vi "Number of Clusters With Silhouette Analysis.vi"() -> ()   [LabVIEW 2020]
doc: "Silhouette analysis can be used to study the separation distance between the resulting clusters. The silhouette plot displays a measure of how close each point in one cluster is to points in the neighboring clusters and thus provides a way to assess parameters like number of clusters visually. This measure has a range of [-1, 1].\n\nSilhouette coefficients (as these values are referred to as) near +1 indicate that the sample is far away from the neighboring clusters. A value of 0 indicates that the sample is on or very close to the decision boundary between two neighboring clusters and negative values indicate that those samples might have been assigned to the wrong cluster.\n\nIn this example the silhouette analysis is used to choose an optimal value for n_clusters. The silhouette plot shows that the n_clusters value of 3, 5 and 6 are a bad pick for the given data due to the presence of clusters with below average silhouette scores and also due to wide fluctuations in the size of the silhouette plots. Silhouette analysis is more ambivalent in deciding between 2 and 4.\n\nAlso from the thickness of the silhouette plot the cluster size can be visualized. The silhouette plot for cluster 0 when n_clusters is equal to 2, is bigger in size owing to the grouping of the 3 sub clusters into one big cluster. However when the n_clusters is equal to 4, all the plots are more or less of similar thickness and hence are of similar sizes as can be also verified from the labelled scatter plot on the right."
uses:
  Model/Unsupervised/Cluster/KMeans/Controls/kmeans_params.ctl
  Display/_Controls/Style.ctl
  Display/Classification/2D/Predicted/Controls/PredictedParameter.ctl
  Model/Unsupervised/Cluster/KMeans/KMeans.lvclass
  C:/Users/cipop/TDF Dropbox/2_Technologies de France/1 - Services et Etudes/PLAIY/2 - DEV/PLAIYLAB/code/Model/Model.lvclass
  Model/Unsupervised/Cluster/KMeans/KMeans.vi
  Preproc/Objet/3 - Model selection and evaluation/3.3 - Metrics and scoring/silhouette_score/Silhouette_Score.vi
  Preproc/Objet/3 - Model selection and evaluation/3.3 - Metrics and scoring/silhouette_samples/Silhouette_Samples.vi
panel:
  out "XY Graph 10":cluster{"X":dbl[], "Y":dbl[]}[](graph)
  out "XY Graph 9":cluster{"X":dbl[], "Y":dbl[]}[](graph)
  out "XY Graph 8":cluster{"X":dbl[], "Y":dbl[]}[](graph)
  out "XY Graph 7":cluster{"X":dbl[], "Y":dbl[]}[](graph)
  out "XY Graph 6":cluster{"X":dbl[], "Y":dbl[]}[](graph) caption="The visualization of the clustered data"
  out "XY Graph 5":cluster{"X":dbl[], "Y":dbl[]}[](graph)
  out "XY Graph 4":cluster{"X":dbl[], "Y":dbl[]}[](graph)
  out "XY Graph 3":cluster{"X":dbl[], "Y":dbl[]}[](graph)
  out "XY Graph 2":cluster{"X":dbl[], "Y":dbl[]}[](graph)
  out "XY Graph":cluster{"X":dbl[], "Y":dbl[]}[](graph) caption="The silhouette plot for the various clusters"
  out "silhouette_avg":string[](array[string])
  in  "Local":T1
  out "error out":errorcluster
  in  "error in":errorcluster
  # "Silhouette analysis for KMeans clustering on sample data with n_cluster = 2"
  # "Silhouette analysis for KMeans clustering on sample data with n_cluster = 3"
  # "Silhouette analysis for KMeans clustering on sample data with n_cluster = 4"
  # "Silhouette analysis for KMeans clustering on sample data with n_cluster = 5"
  # "Silhouette analysis for KMeans clustering on sample data with n_cluster = 6"
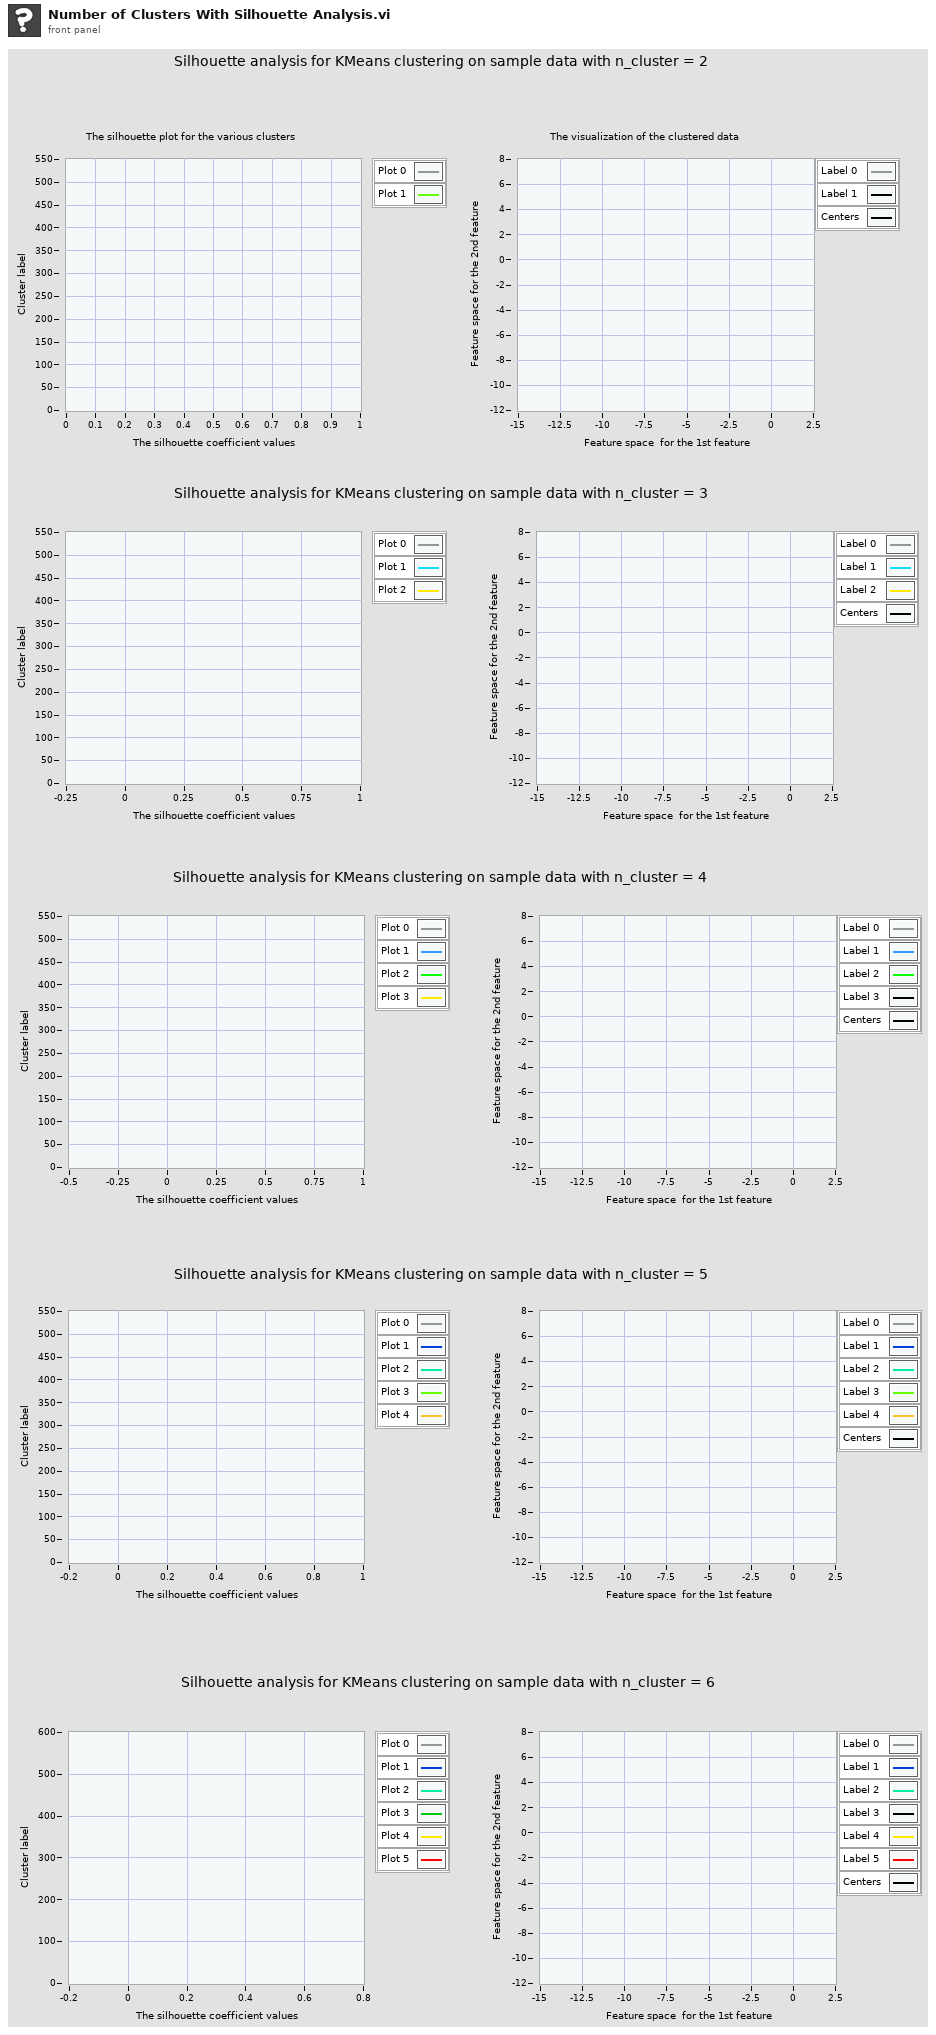
[diagram p1: front panel]
types:
  T1 = cluster{"X":dbl[][], "cluster_labels":dbl[][][], "cluster_centers_":dbl[][][], "sample_silhouette_values":dbl[][], "range_n_clusters":i32[], "ith_cluster_silhouette_values":cluster{"X":dbl[]}[], "y":cluster{"y":dbl[]}[], "i":i32[][][], "Silhouette Plot":refnum<vi>[], "Clustered Plot":refnum<vi>[]}
  T2 = cluster{"n_samples":i32[], "n_features":u32, "centers":i32[][], "cluster_std":dbl[], "centermin":dbl, "centermax":dbl, "shuffle":bool, "random_state":i32, "Returns":string}
  T3 = typedef "kmeans_params.ctl" = cluster{"n_clusters":dbl, "init":cluster{"init_type":string, "init_list":dbl[][]}, "n_init":dbl, "max_iter":dbl, "tol":dbl, "verbose":dbl, "random_state":dbl, "copy_x":bool, "algorithm":string}
  T4 = typedef "Style.ctl" = enum16{"Empty circle", "Full circle", "Empty square", "Full square", "Cross"}
  T5 = typedef "PredictedParameter.ctl" = cluster{"Plot":refnum<vi>, "Data":cluster{"X":dbl[][], "Predict":dbl[][]}, "Indexe":cluster{"X":i32, "Y":i32}, "Point Property":cluster{"Style":T4, "Label Color":u32[]}}
  T6 = cluster{" 4DArray":cluster{"1":string[][], "2":string[][]}[], " 3DArray":cluster{"Tableau":string[][]}[], "Sparse Matrix 2DArray":string[][], " 2DArray":string[][], " 1DArray":string[]}
  T7 = typedef "kmeans_attributes.ctl" = cluster{"cluster_centers_":dbl[][], "labels_":dbl[], "inertia_":dbl, "n_iter_":dbl}
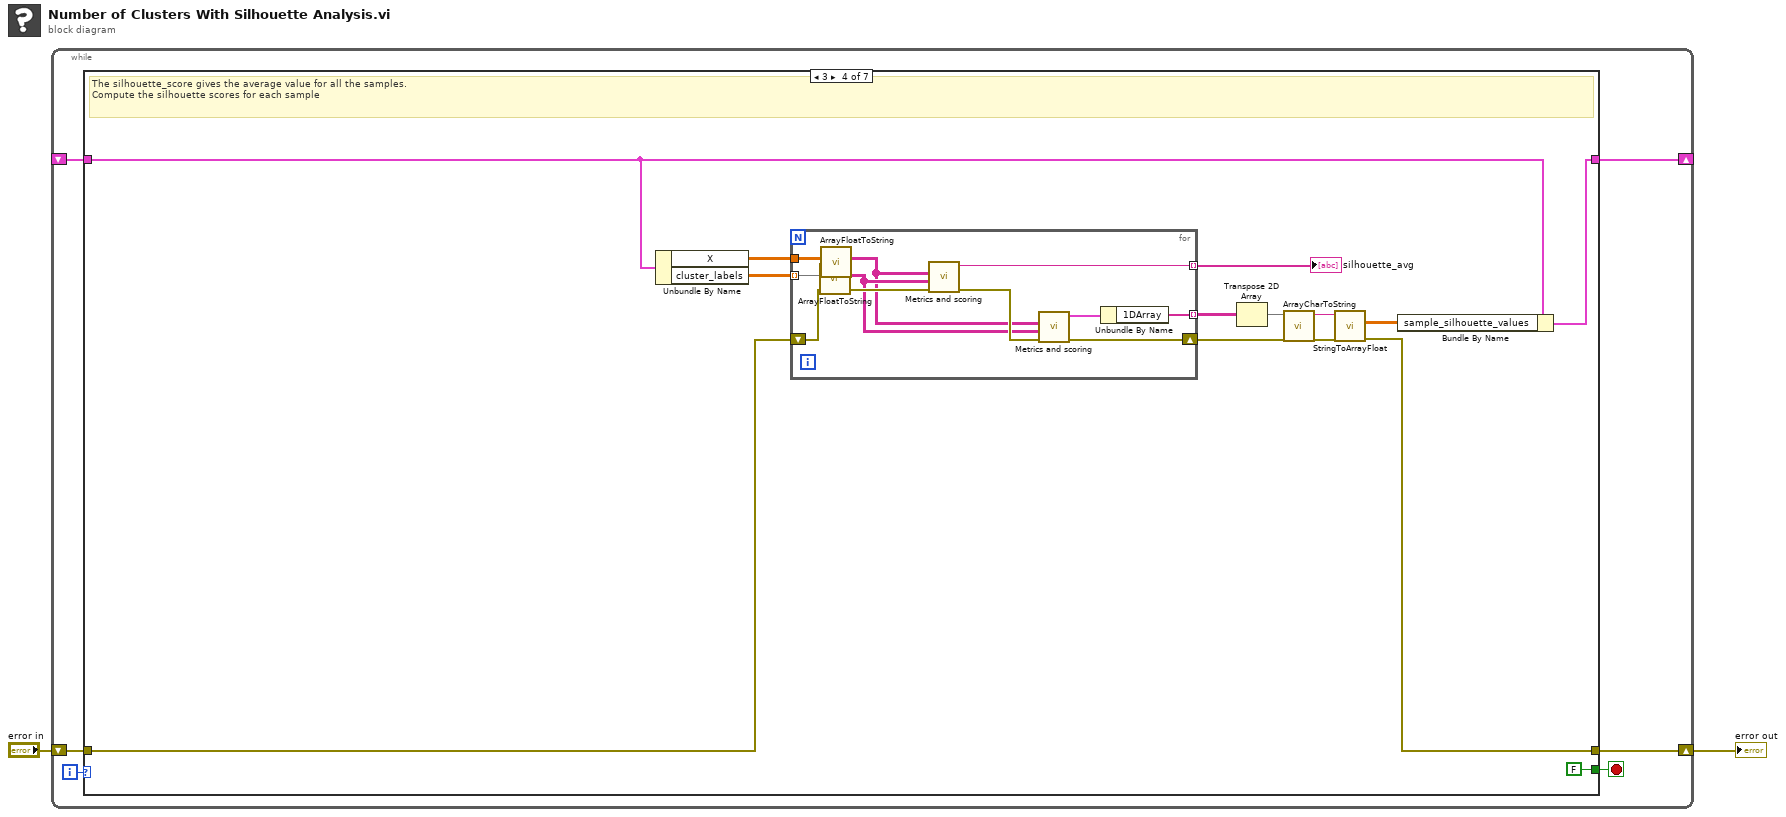
[diagram p0: block diagram]
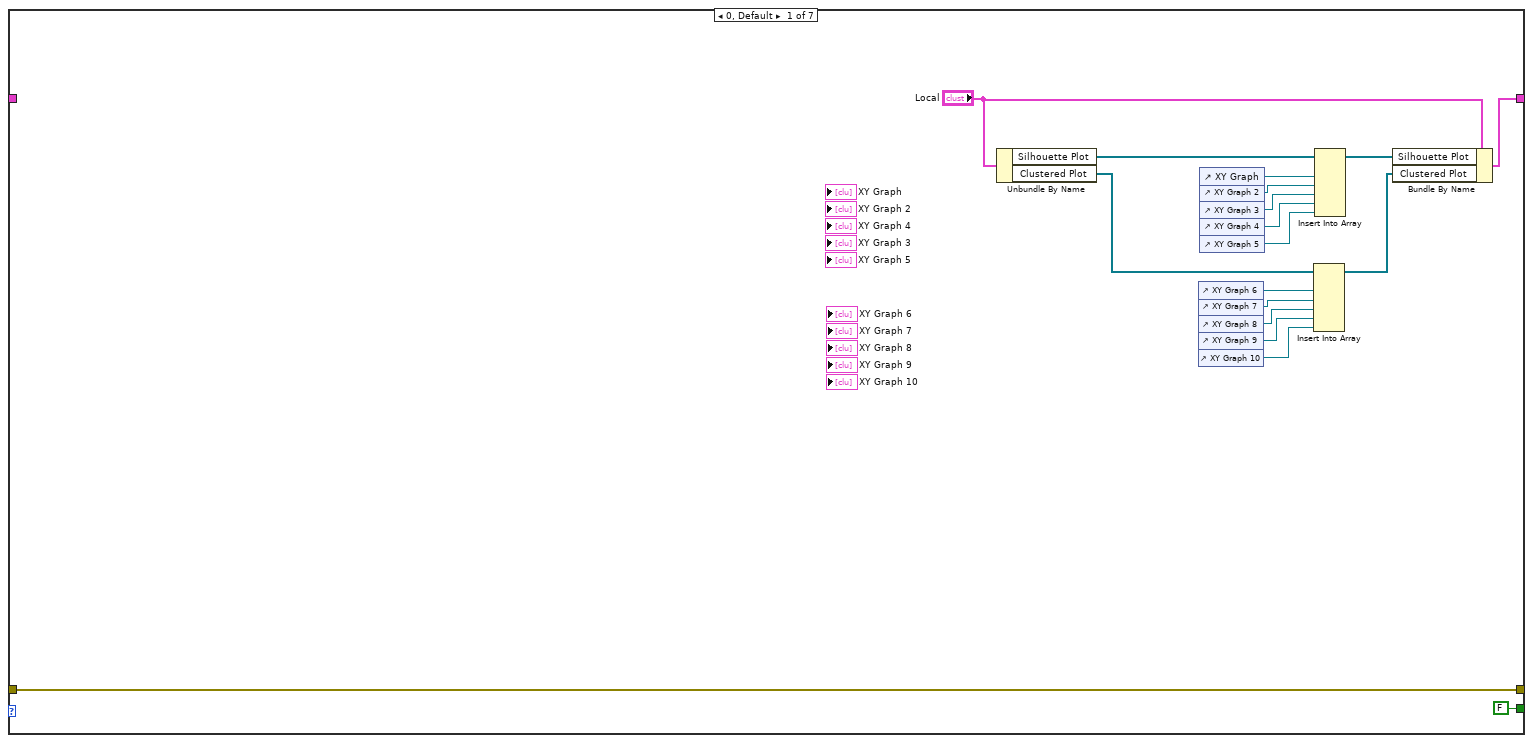
[diagram p2: hidden frame]
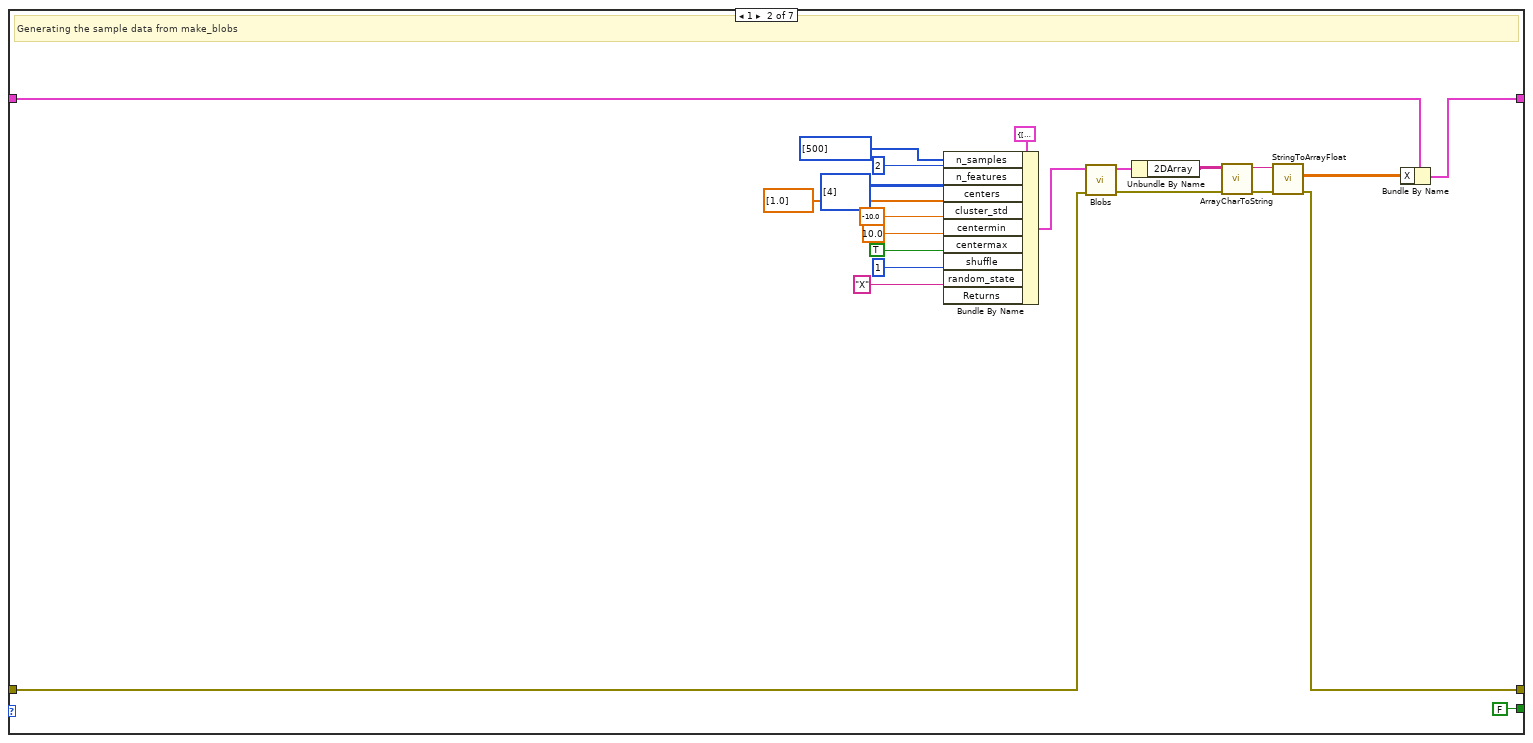
[diagram p3: hidden frame]
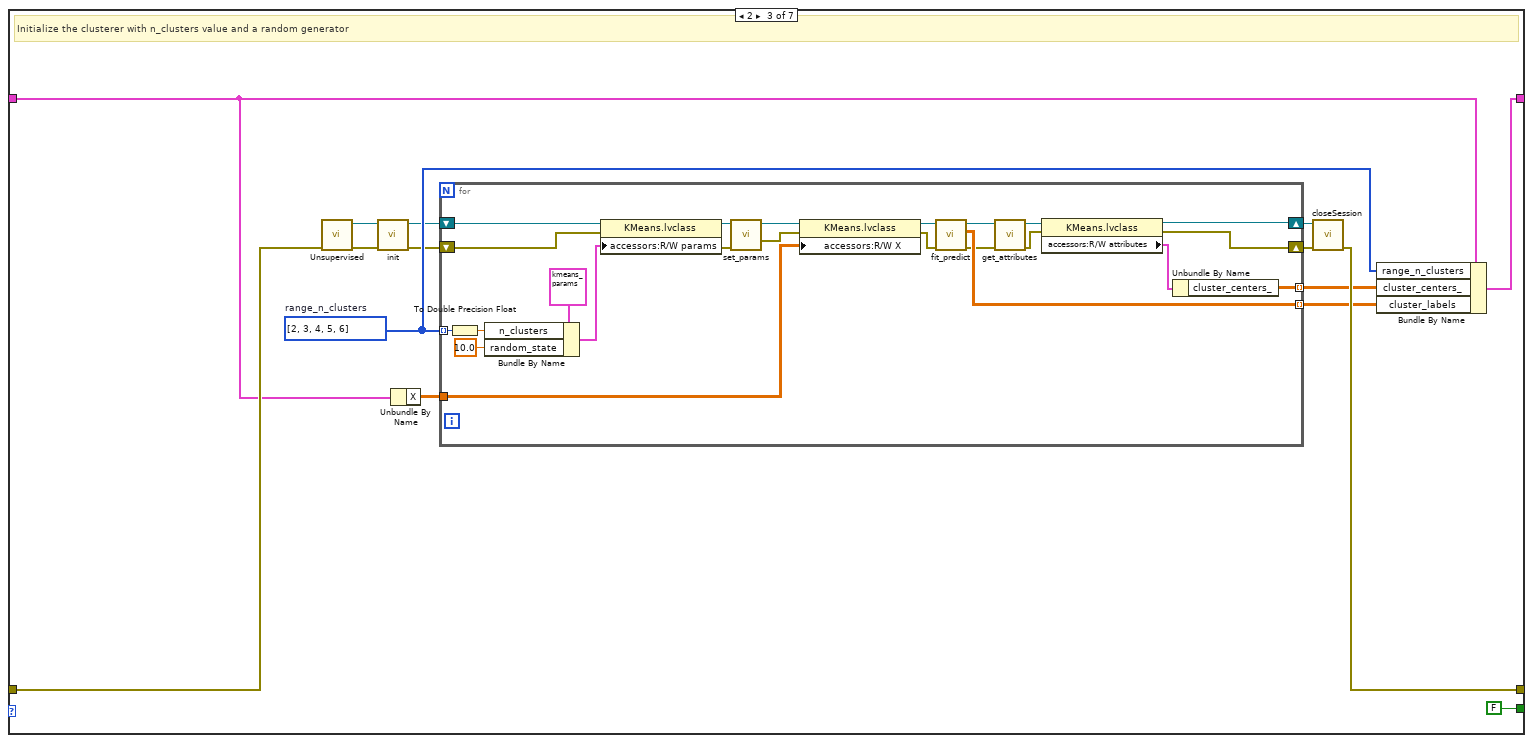
[diagram p4: hidden frame]
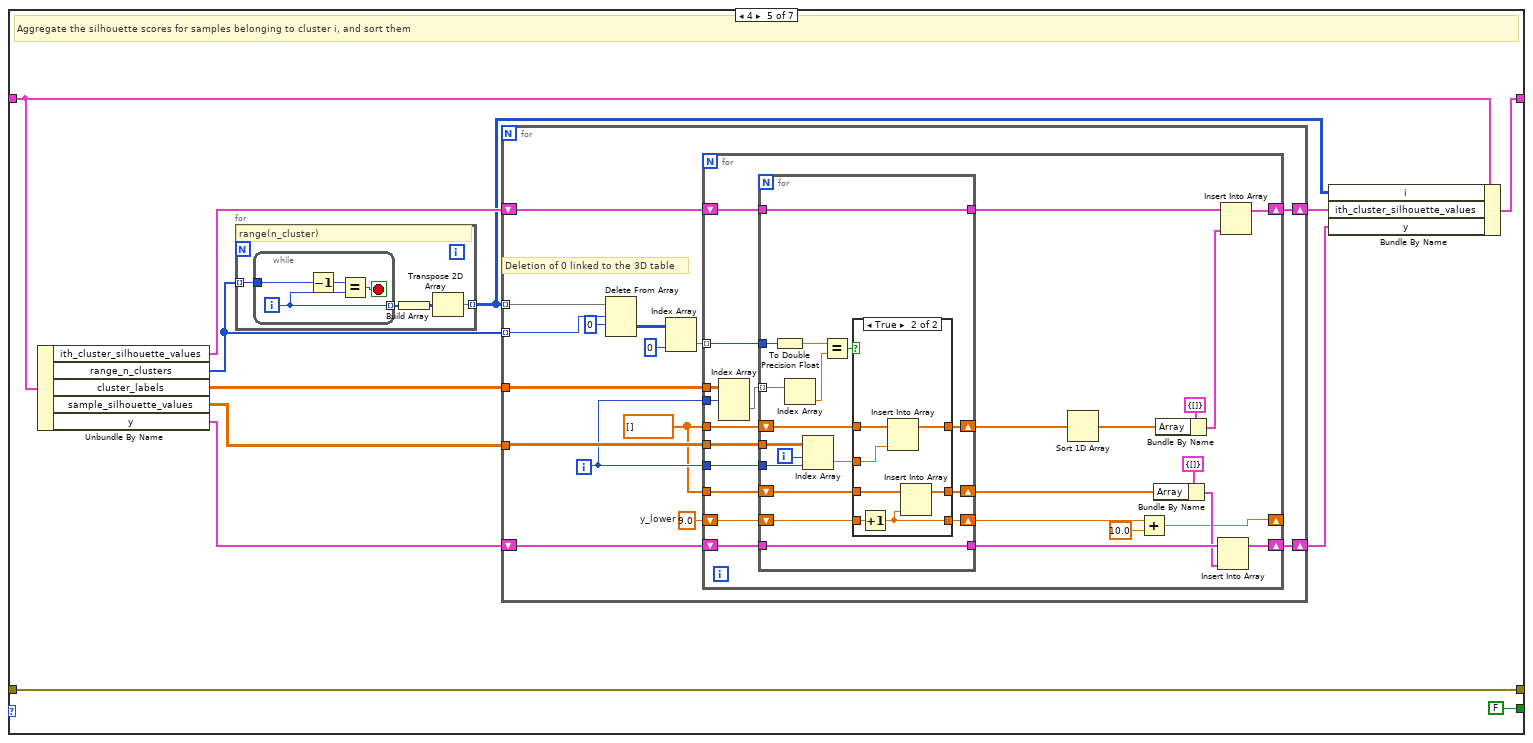
[diagram p5: hidden frame]
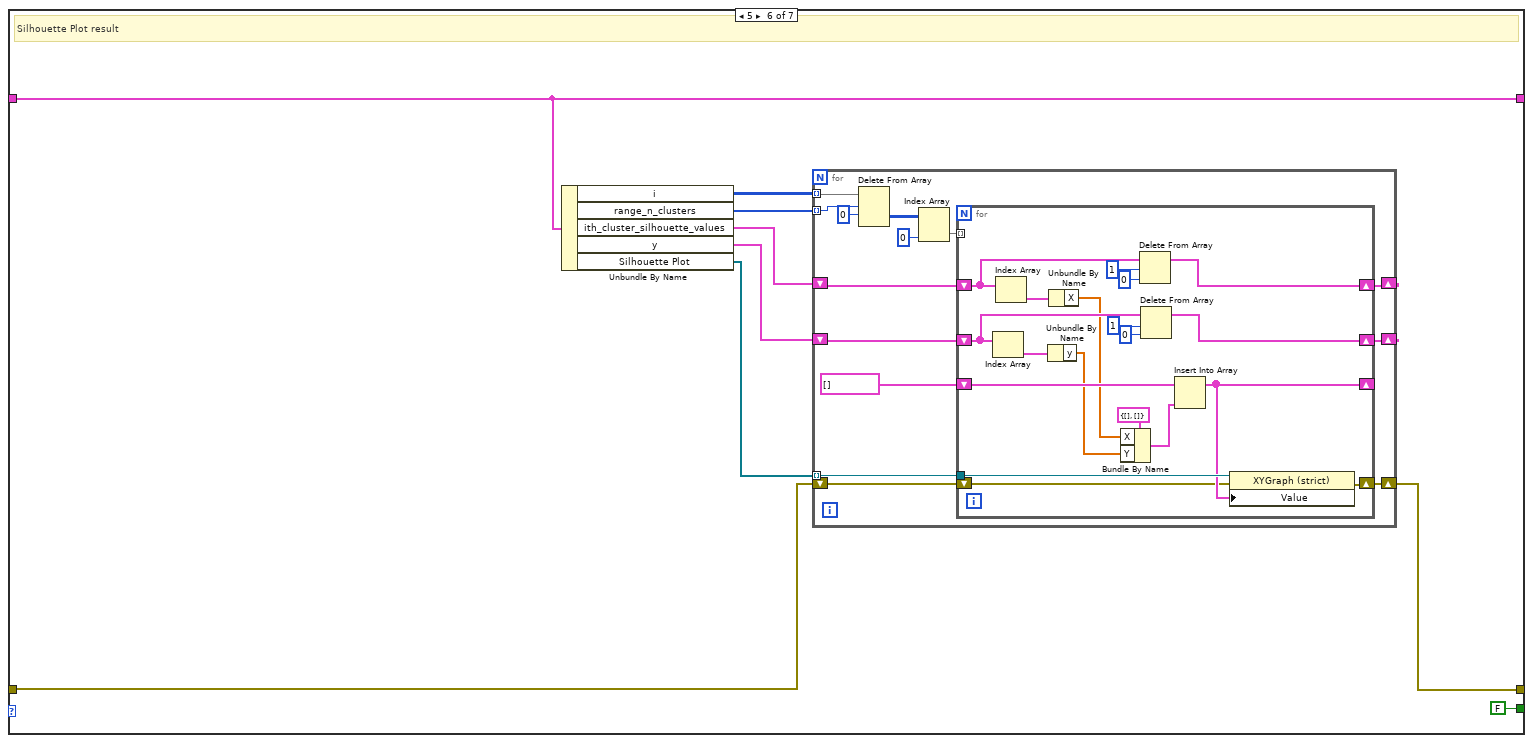
[diagram p7: hidden frame]
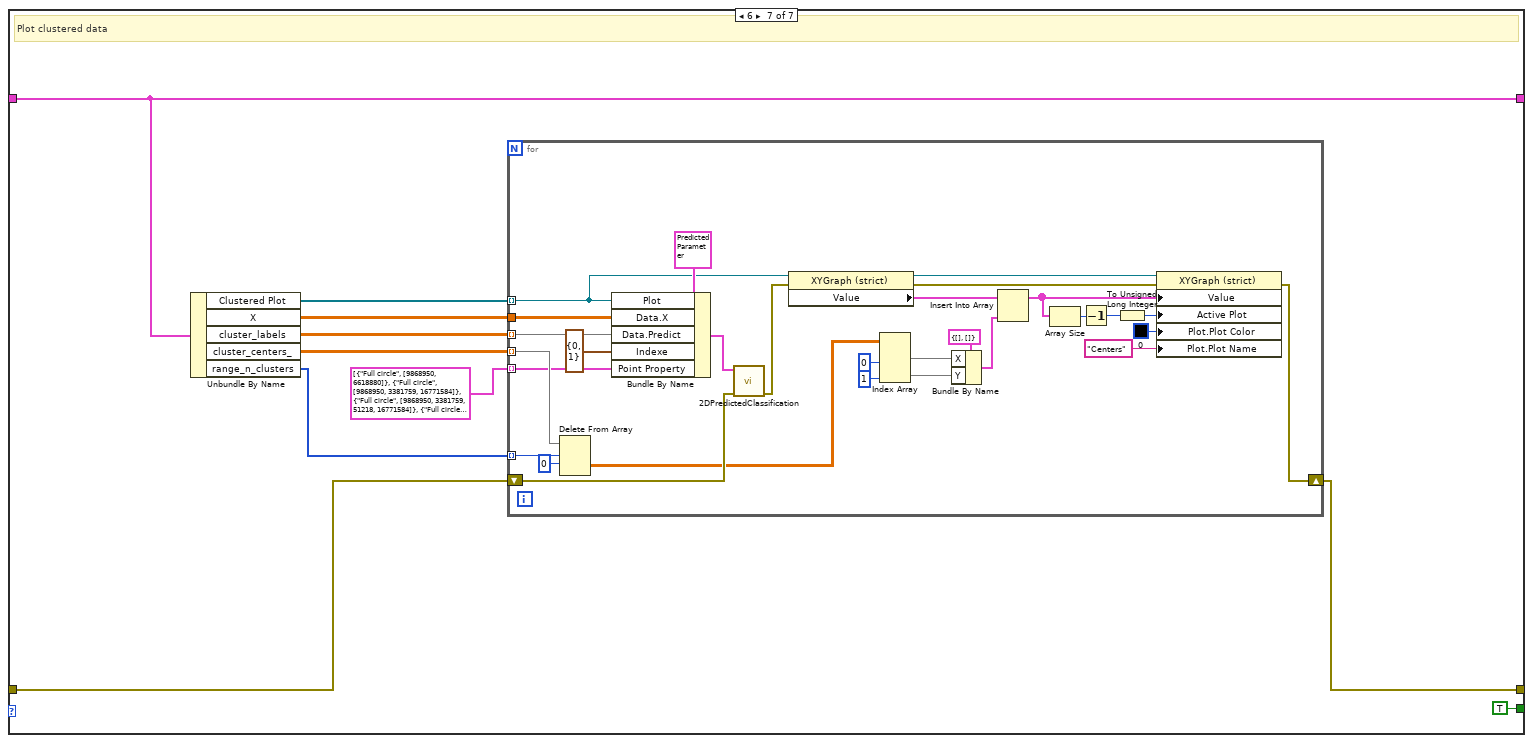
[diagram p8: hidden frame]
diagram:
  n1 = while {
    shift-right: [w6] -> w1
    shift-left: "error in" -> [w7]
    shift-right: [w5] -> _
    shift-left: _ -> [w4]
    i -> [w8]
    stop <- w3 stop-if-true
    n2 = case shown="3" w8 {
      tunnel: w7 -> [w26 w34 w62 w98 w119 w198 w241]
      tunnel: [w26 w33 w61 w94 w119 w197 w240] -> w6
      tunnel: [w21 w31 w59 w95 w113 w203 w246] -> w5
      tunnel: w4 -> [_ w32 w49 w96 w112 w203 w246]
      tunnel: [FALSE FALSE FALSE FALSE FALSE FALSE TRUE] -> w3
      frame 0, Default {
        n3 = Unbundle By Name("Local") -> ("Silhouette Plot"=w23:refnum<vi>[], "Clustered Plot"=w15:refnum<vi>[])
        n4 = control-ref of="XY Graph 6"() -> (w13:refnum<vi>)
        n5 = control-ref of="XY Graph 7"() -> (w12:refnum<vi>)
        n6 = control-ref of="XY Graph 8"() -> (w11:refnum<vi>)
        n7 = control-ref of="XY Graph 9"() -> (w10:refnum<vi>)
        n8 = control-ref of="XY Graph 10"() -> (w9:refnum<vi>)
        n9 = control-ref of="XY Graph"() -> (w20:refnum<vi>)
        n10 = control-ref of="XY Graph 2"() -> (w19:refnum<vi>)
        n11 = control-ref of="XY Graph 3"() -> (w18:refnum<vi>)
        n12 = control-ref of="XY Graph 4"() -> (w17:refnum<vi>)
        n13 = control-ref of="XY Graph 5"() -> (w16:refnum<vi>)
        n14 = Insert Into Array(array=w15, new element #1=w13, new element #2=w12, new element #3=w11, new element #4=w10, new element #5=w9) -> (w14:refnum<vi>[])  [unwired: 1 in]
        n15 = Insert Into Array(array=w23, new element #1=w20, new element #2=w19, new element #3=w18, new element #4=w17, new element #5=w16) -> (w22:refnum<vi>[])  [unwired: 1 in]
        n16 = Bundle By Name(cluster="Local", "Silhouette Plot"=w22, "Clustered Plot"=w14) -> (w21:T1)
      }
      frame 1 {
        # "Generating the sample data from make_blobs"
        n17 = Bundle By Name(cluster=T2 {"n_samples"=[100], "n_features"=2, "centers"=[], "cluster_std"=[1.0], "centermin"=-10.0, "centermax"=10.0, "shuffle"=TRUE, "random_state"=-1, "Returns"="X"} ("make_blobs"), "n_samples"=i32[] [500], "n_features"=u32 2, "centers"=i32[][] [[4]], "cluster_std"=dbl[] [1.0], "centermin"=-10.0, "centermax"=10.0, "shuffle"=TRUE, "random_state"=1, "Returns"="X") -> (w46:T2)
        n18 = call "Blobs.vi"("error in (no error)"=w34, "make_blobs"=w46) -> ("error out"=w35:errorcluster, "Data"=w27:T6)  [unwired: 8 in]
        n19 = Unbundle By Name(w27) -> ("2DArray"=w43:string[][])
        n20 = call "ArrayCharToString.vi"("TAB"=w43) -> ("Instruction"=w47:string)  [unwired: 10 in]
        n21 = call "StringToArrayFloat.vi"("entrée d'erreur (pas d'erreur)"=w35, "Return value"=w47) -> ("error IO"=w33:errorcluster, "2DArray"=w28:dbl[][])  [unwired: 7 in, 1 out]
        n22 = Bundle By Name(cluster=w32, "X"=w28) -> (w31:T1)
      }
      frame 2 {
        w56 = i32[] [2, 3, 4, 5, 6]  # range_n_clusters
        # "Initialize the clusterer with n_clusters value and a random generator"
        n23 = call-poly "Unsupervised.vi"("error in"=w62) -> ("error out"=w52:errorcluster, "out"=w53:refnum<class "KMeans.lvclass">)  [unwired: 9 in]
        n24 = call-dynamic "init.vi"("error in (no error)"=w52, "Model en entrée"=w53) -> ("error out"=w54:errorcluster, "Model en sortie"=w55:refnum<class "KMeans.lvclass">)  [unwired: 8 in]
        n25 = Unbundle By Name(w49) -> ("X"=w60:dbl[][])
        n26 = for {
          tunnel: w60 -> [w75]
          shift-right: [w66] -> w51
          shift-left: w55 -> [w84]
          shift-right: [w65] -> w50
          shift-left: w54 -> [w81]
          tunnel: [w74] -> w58 mode=indexing
          tunnel: w56 -> [w71] mode=indexing
          tunnel: [w63] -> w48 mode=indexing
          n27 = To Double Precision Float(number=w71) -> (double precision float=w73:dbl)
          n28 = Bundle By Name(cluster=T3 {"n_clusters"=8.0, "init"={"init_type"="k-means++", "init_list"=[]}, "n_init"=10.0, "max_iter"=300.0, "tol"=0.0001, "verbose"=0.0, "random_state"=0.0, "copy_x"=TRUE, "algorithm"="auto"} ("R/W params"), "n_clusters"=w73, "random_state"=10.0) -> (w77:T3)
          n29 = property class="KMeans.lvclass"(reference=w84, error in=w81, "accessors:R/W params"=w77) -> (reference out=w83:refnum<class "KMeans.lvclass">, error out=w85:errorcluster)
          n30 = call-dynamic "set_params.vi"("error in (no error)"=w85, "KMeans.lvclass 2"=w83) -> ("error out"=w72:errorcluster, "KMeans.lvclass"=w82:refnum<class "KMeans.lvclass">)  [unwired: 8 in]
          n31 = property class="KMeans.lvclass"(reference=w82, error in=w72, "accessors:R/W X"=w75) -> (reference out=w79:refnum<class "KMeans.lvclass">, error out=w78:errorcluster)
          n32 = call-dynamic "fit_predict.vi"("error in (no error)"=w78, "KMeans.lvclass 2"=w79) -> ("error out"=w67:errorcluster, "C"=w74:dbl[][], "KMeans.lvclass"=w68:refnum<class "KMeans.lvclass">)  [unwired: 7 in]
          n33 = call-dynamic "get_attributes.vi"("error in (no error)"=w67, "KMeans.lvclass 2"=w68) -> ("error out"=w69:errorcluster, "KMeans.lvclass"=w70:refnum<class "KMeans.lvclass">)  [unwired: 8 in]
          n34 = property class="KMeans.lvclass"(reference=w70, error in=w69) -> (reference out=w66:refnum<class "KMeans.lvclass">, error out=w65:errorcluster, "accessors:R/W attributes"=w64:T7)
          n35 = Unbundle By Name(w64) -> ("cluster_centers_"=w63:dbl[][])
        }
        n36 = call-dynamic "closeSession.vi"("error in"=w50, "Python en entrée"=w51) -> ("error out"=w61:errorcluster)  [unwired: 8 in, 1 out]
        n37 = Bundle By Name(cluster=w49, "range_n_clusters"=w56, "cluster_centers_"=w48, "cluster_labels"=w58) -> (w59:T1)
      }
      frame 3 {
        # "The silhouette_score gives the average value for all the samples.\nCompute the silhouette scores for each sample"
        n38 = Unbundle By Name(w96) -> ("X"=w92:dbl[][], "cluster_labels"=w93:dbl[][][])
        n39 = for {
          tunnel: w93 -> [w107] mode=indexing
          tunnel: w92 -> [w108]
          shift-right: [w104] -> w87
          shift-left: w98 -> [w106]
          tunnel: [w101] -> w91 mode=indexing
          tunnel: [w99] -> w90 mode=indexing
          n40 = call "ArrayFloatToString.vi"("2D Data"=w107) -> ("Array"=w103:string[][])  [unwired: 9 in, 1 out]
          n41 = call "ArrayFloatToString.vi"("2D Data"=w108) -> ("Array"=w102:string[][])  [unwired: 9 in, 1 out]
          n42 = call-poly "Metrics and scoring.vi"("error in (no error)"=w106, "labels"=w103, "X"=w102) -> ("error out"=w105:errorcluster, "Score"=w101:string)  [unwired: 7 in]
          n43 = call-poly "Metrics and scoring.vi"("error in (no error)"=w105, "labels"=w103, "X"=w102) -> ("error out"=w104:errorcluster, "Data"=w100:T6)  [unwired: 7 in]
          n44 = Unbundle By Name(w100) -> ("1DArray"=w99:string[])
        }
        "silhouette_avg" <- w91
        n45 = Transpose 2D Array(2D array=w90) -> (transposed array=w88:string[][])
        n46 = call "ArrayCharToString.vi"("TAB"=w88) -> ("Instruction"=w89:string)  [unwired: 10 in]
        n47 = call "StringToArrayFloat.vi"("entrée d'erreur (pas d'erreur)"=w87, "Return value"=w89) -> ("error IO"=w94:errorcluster, "2DArray"=w86:dbl[][])  [unwired: 7 in, 1 out]
        n48 = Bundle By Name(cluster=w96, "sample_silhouette_values"=w86) -> (w95:T1)
      }
      frame 4 {
        # "Aggregate the silhouette scores for samples belonging to cluster i, and sort them"
        n49 = Unbundle By Name(w112) -> ("ith_cluster_silhouette_values"=w115:cluster{"X":dbl[]}[], "range_n_clusters"=w117:i32[], "cluster_labels"=w118:dbl[][][], "sample_silhouette_values"=w116:dbl[][], "y"=w111:cluster{"y":dbl[]}[])
        n50 = for {
          tunnel: w117 -> [w191] mode=indexing
          tunnel: [w188] -> w109 mode=indexing
          # "range(n_cluster)"
          n51 = while {
            tunnel: w191 -> [w194]
            tunnel: [w193] -> w190 mode=indexing
            i -> [w193]
            stop <- w195 stop-if-true
            n52 = Decrement(x=w194) -> (x-1=w192:i32)
            n53 = Equal?(x=w192, y=w193) -> (x = y?=w195:bool)
          }
          n54 = Build Array(w190) -> (w189:i32[][])
          n55 = Transpose 2D Array(2D array=w189) -> (transposed array=w188:i32[][])
        }
        n56 = for {
          tunnel: w116 -> [w129]
          tunnel: w118 -> [w128]
          tunnel: w109 -> [w135] mode=indexing
          tunnel: w117 -> [w134] mode=indexing
          shift-right: [w125] -> w114
          shift-left: w115 -> [w126]
          shift-right: [w123] -> w110
          shift-left: w111 -> [w124]
          i -> [w127]
          w122 = 9.0  # y_lower
          w121 = dbl[] []
          # "Deletion of 0 linked to the 3D table"
          n57 = Delete From Array(array=w135, length=w134, index (row)=0) -> (deleted portion=w132:i32[][])  [unwired: 1 in, 1 out]
          n58 = Index Array(array=w132, index (col)=0 ("disabled index (col)")) -> (element=w130:i32[])  [unwired: 1 in]
          n59 = for {
            tunnel: w130 -> [w160] mode=indexing
            tunnel: w129 -> [w159]
            tunnel: w128 -> [w156]
            tunnel: w121 -> [w158]
            tunnel: w127 -> [w157]
            tunnel: w127 -> [w154]
            shift-right: [w150] -> w125
            shift-left: w126 -> [w153]
            shift-right: [w144] -> w123
            shift-left: w124 -> [w148]
            shift-right: [w139] -> _
            shift-left: w122 -> [w141]
            tunnel: w121 -> [w140]
            n60 = Index Array(array=w156, index (dim 0)=w154) -> (element=w155:dbl[][])  [unwired: 2 in]
            n61 = for {
              tunnel: w155 -> [w176] mode=indexing
              tunnel: w160 -> [w177]
              tunnel: w159 -> [w171]
              shift-right: [w167] -> w137
              shift-left: w158 -> [w172]
              tunnel: w157 -> [w169]
              tunnel: w153 -> [w168]
              tunnel: [w168] -> w149
              tunnel: [w165] -> w147
              tunnel: w148 -> [w165]
              shift-right: [w163] -> w142
              shift-left: w141 -> [w164]
              shift-right: [w161] -> w143
              shift-left: w140 -> [w162]
              i -> [w166]
              n62 = To Double Precision Float(number=w177) -> (double precision float=w174:dbl)
              n63 = Index Array(array=w176) -> (element=w175:dbl)  [unwired: 1 in]
              n64 = Index Array(array=w171, index (row)=w166, index (col)=w169) -> (element=w170:dbl)
              n65 = Equal?(x=w174, y=w175) -> (x = y?=w173:bool)
              n66 = case shown="True" w173 {
                tunnel: w170 -> [_ w186]
                tunnel: w172 -> [w180 w187]
                tunnel: [w180 w184] -> w167
                tunnel: w164 -> [w179 w185]
                tunnel: [w179 w182] -> w163
                tunnel: w162 -> [w178 w183]
                tunnel: [w178 w181] -> w161
                frame False {
                }
                frame True {
                  n67 = Increment(x=w185) -> (x+1=w182:dbl)
                  n68 = Insert Into Array(array=w187, new element=w186) -> (w184:dbl[])  [unwired: 1 in]
                  n69 = Insert Into Array(array=w183, new element=w182) -> (w181:dbl[])  [unwired: 1 in]
                }
              }
            }
            n70 = Sort 1D Array(array=w137) -> (sorted array=w136:dbl[])
            n71 = Add(x=w142, y=10.0) -> (x+y=w139:dbl)
            n72 = Bundle By Name(cluster=cluster{"Array":dbl[]} {"Array"=[]} ("new element/subarray"), "Array"=w143) -> (w145:cluster{"Array":dbl[]})
            n73 = Bundle By Name(cluster=cluster{"Array":dbl[]} {"Array"=[]} ("new element/subarray"), "Array"=w136) -> (w151:cluster{"Array":dbl[]})
            n74 = Insert Into Array(array=w147, new element=w145) -> (w144:cluster{"y":dbl[]}[])  [unwired: 1 in]
            n75 = Insert Into Array(array=w149, new element=w151) -> (w150:cluster{"X":dbl[]}[])  [unwired: 1 in]
          }
        }
        n76 = Bundle By Name(cluster=w112, "i"=w109, "ith_cluster_silhouette_values"=w114, "y"=w110) -> (w113:T1)
      }
      frame 5 {
        # "Silhouette Plot result"
        n77 = Unbundle By Name(w203) -> ("i"=w202:i32[][][], "range_n_clusters"=w201:i32[], "ith_cluster_silhouette_values"=w200:cluster{"X":dbl[]}[], "y"=w199:cluster{"y":dbl[]}[], "Silhouette Plot"=w196:refnum<vi>[])
        n78 = for {
          tunnel: w202 -> [w215] mode=indexing
          tunnel: w201 -> [w214] mode=indexing
          tunnel: w196 -> [w213] mode=indexing
          shift-right: [w208] -> _
          shift-left: w200 -> [w210]
          shift-right: [w207] -> _
          shift-left: w199 -> [w209]
          shift-right: [w205] -> w197
          shift-left: w198 -> [w206]
          n79 = Delete From Array(array=w215, length=w214, index (row)=0) -> (deleted portion=w217:i32[][])  [unwired: 1 in, 1 out]
          n80 = Index Array(array=w217, index (col)=0 ("disabled index (col)")) -> (element=w212:i32[])  [unwired: 1 in]
          n81 = for {
            tunnel: w213 -> [w234]
            tunnel: w212 -> [_] mode=indexing
            shift-right: [w233] -> w208
            shift-left: w210 -> [w236]
            shift-right: [w232] -> w207
            shift-left: w209 -> [w235]
            shift-right: [w221] -> _
            shift-left: cluster{"X":dbl[], "Y":dbl[]}[] [] ("XY Graph 5") -> [w237]
            shift-right: [w219] -> w205
            shift-left: w206 -> [w220]
            n82 = Index Array(array=w235) -> (element=w230:cluster{"y":dbl[]})  [unwired: 1 in]
            n83 = Index Array(array=w236) -> (element=w231:cluster{"X":dbl[]})  [unwired: 1 in]
            n84 = Unbundle By Name(w230) -> ("y"=w227:dbl[])
            n85 = Unbundle By Name(w231) -> ("X"=w228:dbl[])
            n86 = Bundle By Name(cluster=cluster{"X":dbl[], "Y":dbl[]} {"X"=[], "Y"=[]} ("new element/subarray"), "X"=w228, "Y"=w227) -> (w226:cluster{"X":dbl[], "Y":dbl[]})
            n87 = Delete From Array(array=w236, length=1, index=0) -> (array with subset deleted=w233:cluster{"X":dbl[]}[])  [unwired: 1 out]
            n88 = Delete From Array(array=w235, length=1, index=0) -> (array with subset deleted=w232:cluster{"y":dbl[]}[])  [unwired: 1 out]
            n89 = Insert Into Array(array=w237, new element=w226) -> (w221:cluster{"X":dbl[], "Y":dbl[]}[])  [unwired: 1 in]
            n90 = property class="XYGraph (strict)"(reference=w234, error in=w220, "Value"=w221) -> (error out=w219:errorcluster)  [unwired: 1 out]
          }
        }
      }
      frame 6 {
        # "Plot clustered data"
        n91 = Unbundle By Name(w246) -> ("Clustered Plot"=w245:refnum<vi>[], "X"=w244:dbl[][], "cluster_labels"=w243:dbl[][][], "cluster_centers_"=w242:dbl[][][], "range_n_clusters"=w239:i32[])
        n92 = for {
          tunnel: w245 -> [w256] mode=indexing
          tunnel: w244 -> [w257]
          tunnel: w243 -> [w253] mode=indexing
          tunnel: w242 -> [w251] mode=indexing
          shift-right: [w254] -> w240
          shift-left: w241 -> [w255]
          tunnel: w239 -> [w250] mode=indexing
          tunnel: cluster{"Style":T4, "Label Color":u32[]}[] [{"Style"=enum."Full circle", "Label Color"=[9868950, 6618880]}, {"Style"=enum."Full circle", "Label Color"=[9868950, 3381759, 16771584]}, {"Style"=enum."Full circle", "Label Color"=[9868950, 3381759, 51218, 16771584]}, {"Style"=enum."Full circle", "Label Color"=[9868950, 16860, 61349, 6618880, 16761898]}, {"Style"=enum."Full circle", "Label Color"=[9868950, 16860, 1236479, 51218, 16771584, 16711680]}] ("PointProperty") -> [w249] mode=indexing
          n93 = Delete From Array(array=w251, length=w250, index (row)=0) -> (deleted portion=w248:dbl[][])  [unwired: 1 in, 1 out]
          n94 = Bundle By Name(cluster=T5 {"Plot"=refnum, "Data"={"X"=[], "Predict"=[]}, "Indexe"={"X"=0, "Y"=1}, "Point Property"={"Style"=enum."Full circle", "Label Color"=[8978528, 4367871, 1985280]}} ("Parameters"), "Plot"=w256, "Data.X"=w257, "Data.Predict"=w253, "Indexe"=cluster{"X":i32, "Y":i32} {"X"=0, "Y"=1}, "Point Property"=w249) -> (w265:T5)
          n95 = call "2DPredictedClassification.vi"("error in"=w255, "Parameters"=w265) -> ("error out"=w276:errorcluster)  [unwired: 9 in]
          n96 = property class="XYGraph (strict)"(reference=w256, error in=w276) -> (reference out=w267:refnum<vi>, error out=w271:errorcluster, "Value"=w275:cluster{"X":dbl[], "Y":dbl[]}[])
          n97 = Index Array(array=w248, index (col) #1=0 ("disabled index (col)"), index (col) #2=1 ("index (col)")) -> (element #1=w274:dbl[], element #2=w272:dbl[])  [unwired: 2 in]
          n98 = Bundle By Name(cluster=cluster{"X":dbl[], "Y":dbl[]} {"X"=[], "Y"=[]} ("new element/subarray"), "X"=w274, "Y"=w272) -> (w273:cluster{"X":dbl[], "Y":dbl[]})
          n99 = Insert Into Array(array=w275, new element=w273) -> (w268:cluster{"X":dbl[], "Y":dbl[]}[])  [unwired: 1 in]
          n100 = Array Size(array=w268) -> (size(s)=w270:i32)
          n101 = Decrement(x=w270) -> (x-1=w266:i32)
          n102 = To Unsigned Long Integer(number=w266) -> (unsigned 32bit integer=w269:u32)
          n103 = property class="XYGraph (strict)"(reference=w267, error in=w271, "Value"=w268, "Active Plot"=w269, "Plot.Plot Color"=u32 0, "Plot.Plot Name"="Centers") -> (error out=w254:errorcluster)  [unwired: 1 out]
        }
      }
    }
  }
  "error out" <- w1
